vi "TDMS2TDMLogDataConversion.vi"(8 "error in (no error)":errorcluster, 9 "Original Datatype":string, 10 "New Datatype":string, 11 "Channel Name":string) -> (0 "error out":errorcluster)   [LabVIEW 2020]
doc: "This VI reports in the log text that the source datatype was not supported in the TDM storage format and has been coerced."
uses:
  <vilib>/Utility/tdmsutil.llb/TDMS2TDMLogOperation.ctl
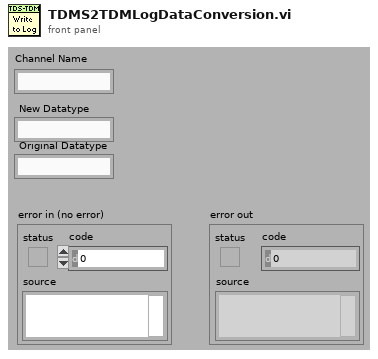
[diagram p1: front panel]
types:
  T1 = typedef "TDMS2TDMLogOperation.ctl" = enum16{"Initialize", "Data Conversion", "Name Conversion", "Write Log File"}
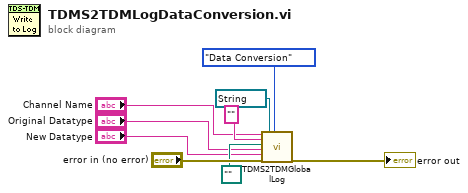
[diagram p0: block diagram]
diagram:
  n1 = call <vilib>:"TDMS2TDMGlobalLog.vi"("Original Name"="Channel Name", "New Name"="" ("Original Name"), "Log File Path"=path "", "Original Datatype"="Original Datatype", "New Datatype"="New Datatype", "error in (no error)"="error in (no error)", "Str Refnum"=refnum<vi> refnum, "Operation"=TDMS2TDMLogOperation."Data Conversion") -> ("error out"=→"error out":errorcluster)  [unwired: 11 in]
